vi "LV86_Get Pixel Value.vi"(4 "Position":cluster{"X":u32, "Y":u32}, 5 "Image In":T1 {"Dialogs" format="%.0b"}) -> (0 "RGB":cluster{"R":u32, "G":u32, "B":u32} {"B" format="%.0x"; "G" format="%.0x"; "R" format="%.0x"}, 1 "I":u32, 2 "Image Out":T1 {"Dialogs" format="%.0b"})   [LabVIEW 2014]
doc: "This VI gets the value of the pixel located at the specified <B>Position</B> and returns its value (either as an 8-bit number or an <B>RGB</B> cluster)."
uses:
  QT_Image.ctl
panel:
  # "This VI gets the value of the pixel located at the specified \nPosition and returns its value (either as an 8-bit \nnumber or an RGB cluster)."
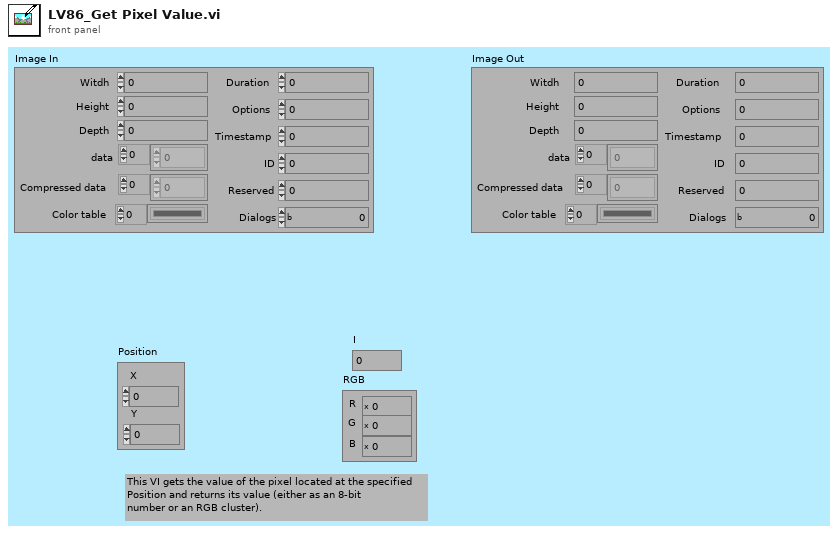
[diagram p1: front panel]
types:
  T1 = typedef "QT_Image.ctl" = cluster{"Witdh":i32, "Height":i32, "Depth":i32, "data":u8[], "Compressed data":u8[], "Color table":u32[], "Duration":i32, "Options":i32, "Timestamp":i32, "ID":i32, "Reserved":i32, "Dialogs":u32}
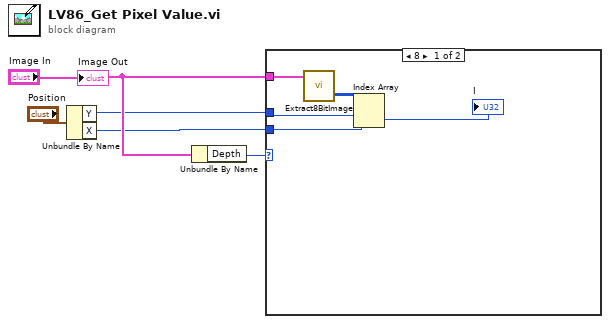
[diagram p0: block diagram]
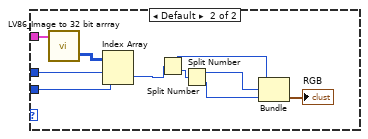
[diagram p2: hidden frame]
diagram:
  n1 = Unbundle By Name("Position") -> ("Y"=w2:u32, "X"=w1:u32)
  n2 = Unbundle By Name("Image In") -> ("Depth"=w4:i32)
  n3 = case shown="8" w4 {
    tunnel: "Image In" -> [w10 w14]
    tunnel: w2 -> [w8 w12]
    tunnel: w1 -> [w7 w11]
    frame 8 {
      n4 = call "Extract8BitImage.vi"("Image in"=w10) -> ("Intensity Graph"=w9:u8[][])  [unwired: 1 in, 1 out]
      n5 = Index Array(array=w9, index (row)=w8, index (col)=w7) -> (element=→"I":u8)
    }
    frame Default {
      n6 = call "LV86_Image to 32 bit arrray.vi"("Image In"=w14) -> ("Intensity Graph"=w15:u32[][])  [unwired: 1 in, 1 out]
      n7 = Index Array(array=w15, index (row)=w12, index (col)=w11) -> (element=w13:u32)
      n8 = Split Number(x=w13) -> (hi(x)=w18:u16, lo(x)=w19:u16)
      n9 = Split Number(x=w19) -> (hi(x)=w17:u8, lo(x)=w16:u8)
      n10 = Bundle(w18, w17, w16) -> (→"RGB":cluster{u16, u8, u8})  [unwired: 1 out]
    }
  }
  "Image Out" <- "Image In"
